vi "Read Dev Auto.vi"(8 "error in (no error)":errorcluster, 11 "VISA resource name":refnum<visa-resource-name>) -> (0 "error out":errorcluster, 2 "dev point auto":T1, 3 "VISA resource name out":refnum<visa-resource-name>)   [LabVIEW 2020, in "Andeen-Hagerling 2700A.lvlib"]
doc: "Return the value of the deviation mode auto parameter.\n\nDuring each initialization of the deviation mode the DUT is\nmeasured resulting in a set of capacitance and loss values\nknown as the Initial Deviation Reading. These values may be\nused to automatically establish new Deviation Setpoint values.\nAlternatively, the Deviation Setpoints remain fixed at\ntheir previous values and the Initial Deviation Readings are\nused simply to verify that the DUT is within the previously\nspecified upper and lower boundaries."
uses:
  Andeen-Hagerling 2700A.lvlib
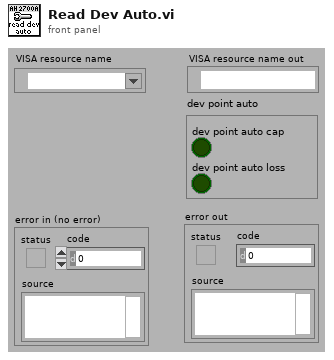
[diagram p1: front panel]
types:
  T1 = cluster{"dev point auto cap":bool, "dev point auto loss":bool}
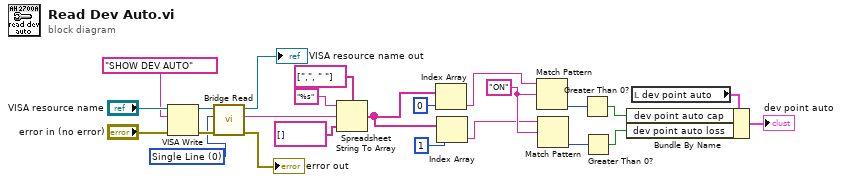
[diagram p0: block diagram]
diagram:
  w1 = u16 0 items=["Single Line", "Multi-Line"] ("Multiline")
  w16 = "ON" ("regular expression")
  n1 = VISA Write(VISA resource name="VISA resource name", write buffer="SHOW DEV AUTO" ("command"), error in (no error)="error in (no error)") -> (VISA resource name out=w6:refnum<visa-resource-name>, error out=w2:errorcluster)  [unwired: 1 out]
  n2 = call "Bridge Read.vi"("error in (no error)"=w2, "multiline"=w1, "VISA resource name"=w6) -> ("error out"=→"error out":errorcluster, "read buffer"=w4:string, "VISA resource name out"=→"VISA resource name out":refnum<visa-resource-name>)  [unwired: 6 in]
  n3 = Spreadsheet String To Array(delimiter (Tab)=string[] [",", " "], format string="%s", spreadsheet string=w4, array type (2D Dbl)=string[] []) -> (array=w17:string[])
  n4 = Index Array(array=w17, index=0) -> (element=w14:string)
  n5 = Index Array(array=w17, index=1) -> (element=w15:string)
  n6 = Match Pattern(string=w14, regular expression=w16) -> (offset past match=w13:i32)  [unwired: 1 in, 3 out]
  n7 = Match Pattern(string=w15, regular expression=w16) -> (offset past match=w12:i32)  [unwired: 1 in, 3 out]
  n8 = Greater Than 0?(x=w13) -> (x > 0?=w9:bool)
  n9 = Greater Than 0?(x=w12) -> (x > 0?=w8:bool)
  n10 = local read "dev point auto"() -> (w10:T1)
  n11 = Bundle By Name(cluster=w10, "dev point auto cap"=w9, "dev point auto loss"=w8) -> (→"dev point auto":T1)
